vi "S-Curve Newton Method Time.vi"(4 "v_f":dbl, 6 "v_i":dbl, 7 "err":dbl, 8 "g":dbl, 9 "j":dbl, 10 "a":dbl, 11 "v":dbl) -> (3 "t_out":dbl)   [LabVIEW 2020]
uses:
  <vilib>/ptbypt/NI_PtbyPt.lvlib
panel:
  out "iterations":i32
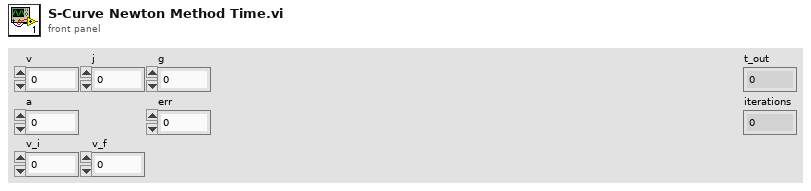
[diagram p1: front panel]
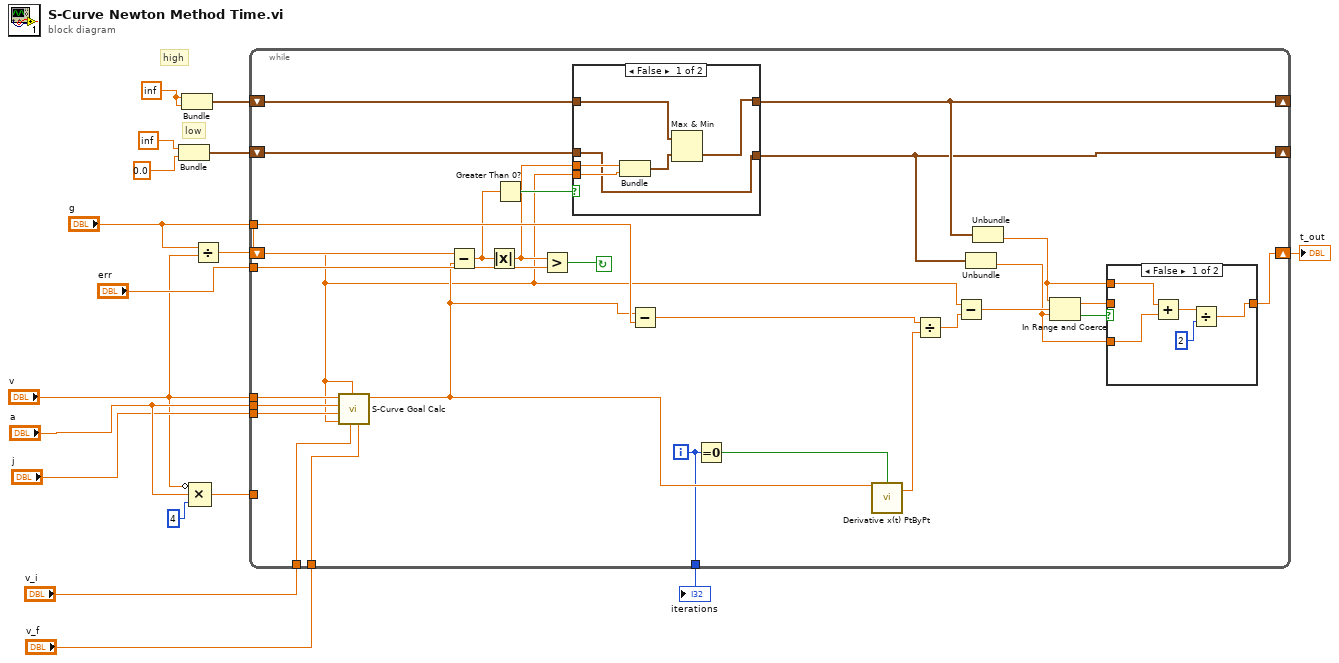
[diagram p0: block diagram]
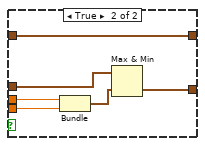
[diagram p3: hidden frame]
diagram:
  w6 = inf
  # "low"
  # "high"
  n1 = Bundle(inf, 0.0) -> (w2:cluster{dbl, dbl})  [unwired: 1 in]
  n2 = Bundle(w6, w6) -> (w5:cluster{dbl, dbl})  [unwired: 1 in]
  n3 = Compound Arithmetic op=MULTIPLY(invert "v", "a", 4) -> (w16:dbl)
  n4 = Divide(x="g", y="v") -> (x/y=w7:dbl)
  n5 = while {
    tunnel: "v" -> [w33]
    tunnel: "a" -> [w45]
    tunnel: "j" -> [w44]
    tunnel: "v_i" -> [w43]
    tunnel: "v_f" -> [w42]
    tunnel: w16 -> [_]
    shift-right: [w21] -> w10
    shift-left: w7 -> [w18]
    tunnel: "g" -> [w38]
    tunnel: "err" -> [w41]
    shift-right: [w26] -> _
    shift-left: w5 -> [w27]
    shift-right: [w25] -> _
    shift-left: w2 -> [w29]
    tunnel: [w24] -> w1
    i -> [w24]
    stop <- w40 continue-if-true
    n6 = call "S-Curve Goal Calc.vi"("v_f"=w42, "v_i"=w43, "x"=w18, "t"=w18, "j"=w44, "a"=w45, "v"=w33) -> ("goal"=w35:dbl)  [unwired: 4 in]
    n7 = Subtract(x=w38, y=w35) -> (x-y=w31:dbl)
    n8 = Absolute Value(x=w31) -> (abs(x)=w28:dbl)
    n9 = Greater Than 0?(x=w31) -> (x > 0?=w30:bool)
    n10 = Greater?(x=w28, y=w41) -> (0:w40:bool)
    n11 = case shown="False" w30 {
      tunnel: w29 -> [w52 w60]
      tunnel: w28 -> [w56 w63]
      tunnel: w18 -> [w55 w62]
      tunnel: [w52 w59] -> w25
      tunnel: w27 -> [w54 w58]
      tunnel: [w53 w58] -> w26
      frame False {
        n12 = Bundle(w56, w55) -> (w57:cluster{dbl, dbl})  [unwired: 1 in]
        n13 = Max & Min(x=w54, y=w57) -> (min(x,y)=w53:cluster{dbl, dbl})  [unwired: 1 out]
      }
      frame True {
        n14 = Bundle(w63, w62) -> (w61:cluster{dbl, dbl})  [unwired: 1 in]
        n15 = Max & Min(x=w60, y=w61) -> (min(x,y)=w59:cluster{dbl, dbl})  [unwired: 1 out]
      }
    }
    n16 = Subtract(x=w35, y=w38) -> (x-y=w37:dbl)
    n17 = Equal To 0?(x=w24) -> (x = 0?=w32:bool)
    n18 = call <vilib>:"Derivative x(t) PtByPt.vi"("initialize"=w32, "x"=w35) -> ("dx/dt"=w34:dbl)  [unwired: 2 in, 1 out]
    n19 = Divide(x=w37, y=w34) -> (x/y=w39:dbl)
    n20 = Subtract(x=w18, y=w39) -> (x-y=w36:dbl)
    n21 = Unbundle(w25) -> (w19:dbl)  [unwired: 1 out]
    n22 = Unbundle(w26) -> (w20:dbl)  [unwired: 1 out]
    n23 = In Range and Coerce(upper limit=w20, x=w36, lower limit=w19) -> (coerced(x)=w22:dbl, In Range?=w23:bool)
    n24 = case shown="False" w23 {
      tunnel: w22 -> [_ w51]
      tunnel: [w46 w51] -> w21
      tunnel: w20 -> [w50 _]
      tunnel: w19 -> [w49 _]
      frame False {
        n25 = Add(x=w50, y=w49) -> (x+y=w48:dbl)
        n26 = Divide(x=w48, y=2) -> (x/y=w46:dbl)
      }
      frame True {
      }
    }
  }
  "t_out" <- w10
  "iterations" <- w1
